vi "File Checksum.vi"   [LabVIEW 2020, in "NI_Message Digest API.lvlib"]
doc: "Computes the message digest on the contents of a file. You must manually select the polymorphic instance you want to use."
uses:
  <vilib>/security/Message Digest/API/NI_Message Digest API.lvlib
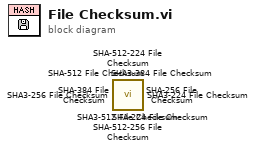
[diagram p0: block diagram]
diagram:
  n1 = call <vilib>:"SHA3-512 File Checksum.vi"() -> ()  [unwired: 10 in, 2 out]
  n2 = call <vilib>:"SHA3-384 File Checksum.vi"() -> ()  [unwired: 10 in, 2 out]
  n3 = call <vilib>:"SHA3-256 File Checksum.vi"() -> ()  [unwired: 10 in, 2 out]
  n4 = call <vilib>:"SHA3-224 File Checksum.vi"() -> ()  [unwired: 10 in, 2 out]
  n5 = call <vilib>:"SHA-512-256 File Checksum.vi"() -> ()  [unwired: 10 in, 2 out]
  n6 = call <vilib>:"SHA-512-224 File Checksum.vi"() -> ()  [unwired: 10 in, 2 out]
  n7 = call <vilib>:"SHA-512 File Checksum.vi"() -> ()  [unwired: 10 in, 2 out]
  n8 = call <vilib>:"SHA-384 File Checksum.vi"() -> ()  [unwired: 10 in, 2 out]
  n9 = call <vilib>:"SHA-256 File Checksum.vi"() -> ()  [unwired: 10 in, 2 out]
  n10 = call <vilib>:"SHA-224 File Checksum.vi"() -> ()  [unwired: 10 in, 2 out]
